vi "CANOpen_SDO_Add error code.vi"(0 "completion code in":u32, 1 "error in (no error)":errorcluster) -> (20 "completion code out":dbl)   [LabVIEW 2013, in "CANOpen Addon Custom Device.lvlib"]
uses:
  CANOpen Addon Custom Device.lvlib
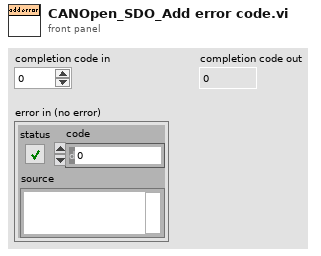
[diagram p1: front panel]
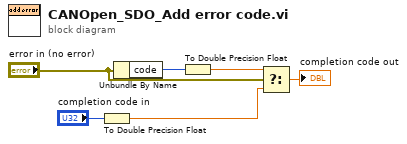
[diagram p0: block diagram]
diagram:
  n1 = To Double Precision Float(number="completion code in") -> (double precision float=w2:dbl)
  n2 = Unbundle By Name("error in (no error)") -> ("code"=w5:i32)
  n3 = To Double Precision Float(number=w5) -> (double precision float=w1:dbl)
  n4 = Select(t=w1, s="error in (no error)", f=w2) -> (s? t:f=→"completion code out":dbl)
